vi "LowLvCtrl_Clear.vi"(8 "error in (no error)":errorcluster, 9 "DAQmx Task Name":refnum<k21>="LoadCells_AI", 10 "FPGA VI Reference In":refnum<k20>) -> (0 "error out":errorcluster)   [LabVIEW 2015]
uses:
  <vilib>/Utility/error.llb/Error Cluster From Error Code.vi
  <vilib>/rvi/errors/niLvFpgaAdjustHostInterfaceError.vi
  <vilib>/FPGAPlugInAG/Dynamic/niLvFpga_Close_Dynamic.vi
  <vilib>/rvi/interface/nirviReadWriteControl/nirviReadWriteControl.xnode
  <vilib>/rvi/interface/nirviCloseFPGA/nirviCloseFPGA.xnode
  NiFpgaLv.dll
  <vilib>/rvi/interface/Simulation/niFpgaSimulationCallBeginRW.vi
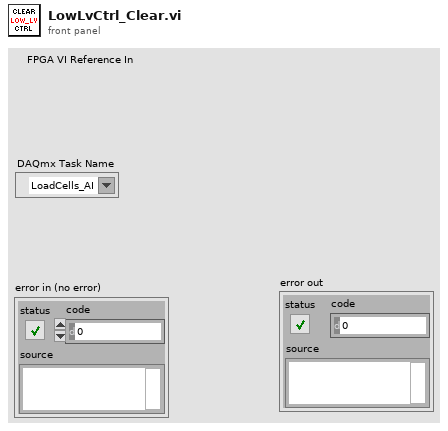
[diagram p1: front panel]
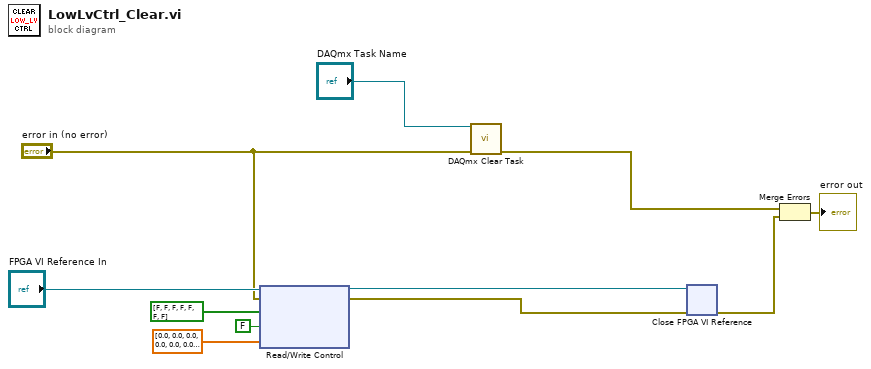
[diagram p0: block diagram]
diagram:
  n1 = xnode "Read/Write Control"("FPGA VI Reference In"="FPGA VI Reference In", "error in"="error in (no error)", "Enable"=bool[] [FALSE, FALSE, FALSE, FALSE, FALSE, FALSE, FALSE], "EnableMaster"=FALSE, "AmpCmd"=sgl[] [0.0, 0.0, 0.0, 0.0, 0.0, 0.0, 0.0]) -> ("FPGA VI Reference Out"=w3:refnum<k20>, "error out"=w4:errorcluster)
  n2 = call <vilib>:"DAQmx Clear Task.vi"("task in"="DAQmx Task Name", "error in"="error in (no error)") -> ("error out"=w5:errorcluster)  [unwired: 13 in]
  n3 = xnode "Close FPGA VI Reference"("FPGA VI Reference In"=w3, "error in"=w4) -> ("error out"=w2:errorcluster)
  n4 = Merge Errors(w5, w2) -> (→"error out":errorcluster)
